vi "Voltage Write Array.vi"(10 "Voltage.AV":dbl[](array[numeric]), 11 "Device in":refnum<class "Device.lvclass">) -> (3 "Device out":refnum<class "Device.lvclass">)   [LabVIEW 2023, in "Device.lvclass"]
uses:
  Device.lvclass
  Device.lvclass/Device.ctl
  Low Level Capabilities/Voltage/Voltage Actual Value/Voltage Actual Value.lvclass
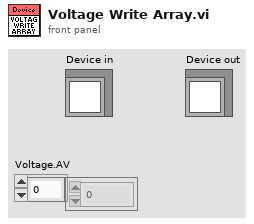
[diagram p1: front panel]
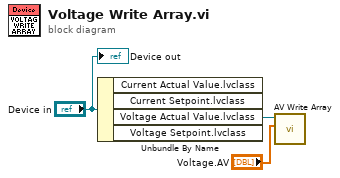
[diagram p0: block diagram]
diagram:
  n1 = Unbundle By Name("Device in") -> ("Voltage Actual Value.lvclass"=w2:refnum<class "Voltage Actual Value.lvclass">)  [unwired: 3 out]
  n2 = call-dynamic "AV Write Array.vi"("Actual Value"="Voltage.AV", "Voltage Actual Value in"=w2) -> ()  [unwired: 8 in, 2 out]
  "Device out" <- "Device in"
